vi "test - Module Name Case Insensitive.vi"(8 "error in (no error)":errorcluster, 11 "TestCase in":refnum<class "testcase-Basic-Function.lvclass">) -> (0 "error out":errorcluster, 3 "TestCase out":refnum<class "testcase-Basic-Function.lvclass">)   [LabVIEW 2017, in "testcase-Basic-Function.lvclass"]
uses:
  testcase-Basic-Function.lvclass
  testcase-Basic-Function.lvclass/testcase-Basic-Function.ctl
  src/user.lib/_NEVSTOP/Communicable State Machine(CSM)/_Support/Typedef/_CSM_MODE.ctl
  <vilib>/addons/_JKI Toolkits/VI Tester/TestCase.llb/TestCase.lvclass
  src/user.lib/_NEVSTOP/Communicable State Machine(CSM)/Communicable State Machine.lvlib
  C:/Program Files (x86)/National Instruments/LabVIEW 2017/vi.lib/addons/_JKI Toolkits/VI Tester/TestCase.llb/TestCase.lvclass
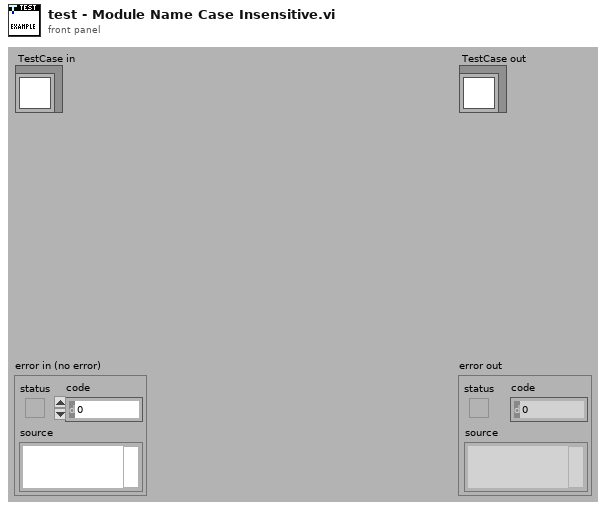
[diagram p1: front panel]
types:
  T1 = typedef "Communicable State Machine.lvlib/_CSM_MODE.ctl" = enum16{"Not Exist", "Stand Alone", "CSM", "Worker", "Worker Agent", "Chain Node", "Chain"}
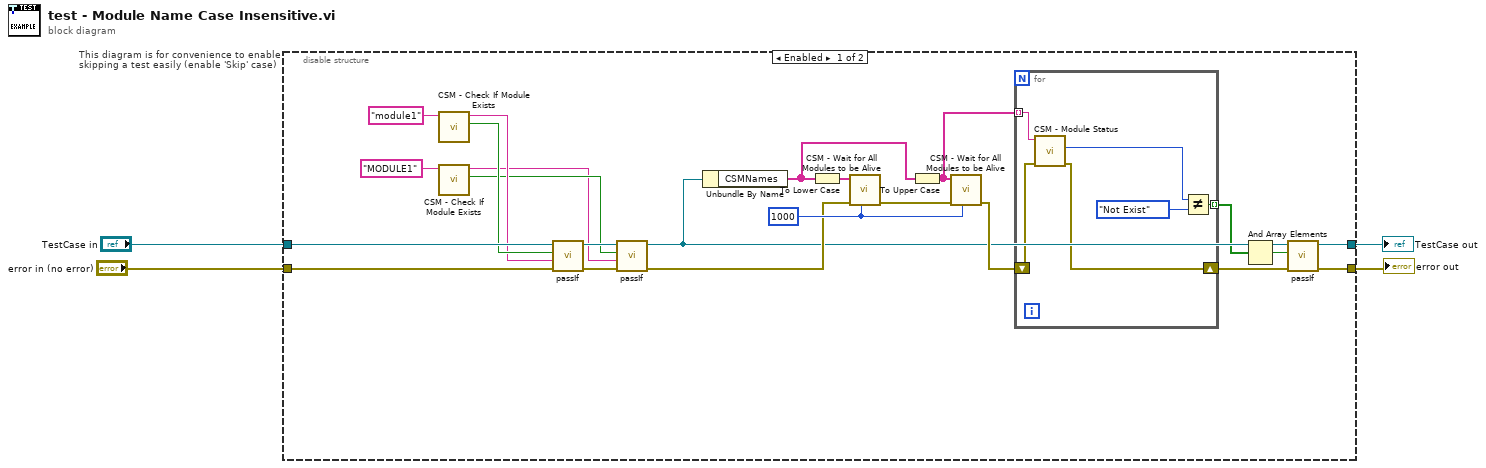
[diagram p0: block diagram]
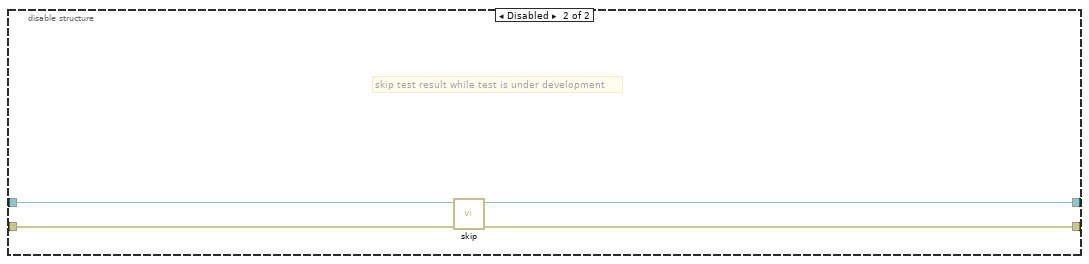
[diagram p2: hidden frame]
diagram:
  n1 = disable-structure "This diagram is for convenience to enable skipping a test easily (enable 'Skip' case)" shown="Enabled" {
    disable-tunnel: "TestCase in" -> [w27 w37]
    disable-tunnel: [w10 w35] -> w1
    disable-tunnel: [w9 w36] -> w3
    disable-tunnel: "error in (no error)" -> [w26 w34]
    frame Enabled {
      w17 = u32 1000 ("Timeout(5000 ms)")
      n2 = call "CSM - Check If Module Exists.vi"("CSM Name"="module1") -> ("Exist?"=w23:bool, "CSM Name (Dup)"=w22:string)  [unwired: 8 in, 1 out]
      n3 = call "CSM - Check If Module Exists.vi"("CSM Name"="MODULE1") -> ("Exist?"=w19:bool, "CSM Name (Dup)"=w18:string)  [unwired: 8 in, 1 out]
      n4 = call-dynamic "passIf.vi"("error in (no error)"=w26, "message (\"\")"=w22, "pass"=w23, "TestCase in"=w27) -> ("error out"=w21:errorcluster, "TestCase out"=w20:refnum<class "testcase-Basic-Function.lvclass">)  [unwired: 6 in]
      n5 = call-dynamic "passIf.vi"("error in (no error)"=w21, "message (\"\")"=w18, "pass"=w19, "TestCase in"=w20) -> ("error out"=w15:errorcluster, "TestCase out"=w11:refnum<class "testcase-Basic-Function.lvclass">)  [unwired: 6 in]
      n6 = Unbundle By Name(w11) -> ("CSMNames"=w16:string[])
      n7 = To Lower Case(string=w16) -> (all lower case string=w13:string[])
      n8 = call "CSM - Wait for All Modules to be Alive.vi"("Timeout (5000 ms)"=w17, "Error In"=w15, "CSM Names"=w13) -> ("error out"=w14:errorcluster)  [unwired: 6 in, 2 out]
      n9 = To Upper Case(1:w16) -> (0:w5:string[])
      n10 = call "CSM - Wait for All Modules to be Alive.vi"("Timeout (5000 ms)"=w17, "Error In"=w14, "CSM Names"=w5) -> ("error out"=w12:errorcluster)  [unwired: 6 in, 2 out]
      n11 = for {
        tunnel: w5 -> [w32] mode=indexing
        tunnel: [w28] -> w7 mode=indexing
        shift-right: [w31] -> w8
        shift-left: w12 -> [w33]
        n12 = call "CSM - Module Status.vi"("Error In"=w33, "CSM Name"=w32) -> ("error out"=w31:errorcluster, "Mode"=w30:T1)  [unwired: 5 in, 3 out]
        n13 = Not Equal?(x=w30, y=_CSM_MODE."Not Exist") -> (x != y?=w28:bool)
      }
      n14 = And Array Elements(Boolean array=w7) -> (logical AND=w6:bool)
      n15 = call-dynamic "passIf.vi"("error in (no error)"=w8, "pass"=w6, "TestCase in"=w11) -> ("error out"=w9:errorcluster, "TestCase out"=w10:refnum<class "testcase-Basic-Function.lvclass">)  [unwired: 7 in]
    }
    frame Disabled {
      # "skip test result while test is under development"
      n16 = call <vilib>:"skip.vi"("error in (no error)"=w34, "TestCase in"=w37) -> ("error out"=w36:errorcluster, "TestCase out"=w35:refnum<class "testcase-Basic-Function.lvclass">)  [unwired: 8 in]
    }
  }
  "error out" <- w3
  "TestCase out" <- w1
